vi "Set Controls.vi"(1 "Disabled Controls":refnum<vi>[](array[refnum]), 2 "Enabled Controls":refnum<vi>[](array[refnum])) -> ()   [LabVIEW 2017]
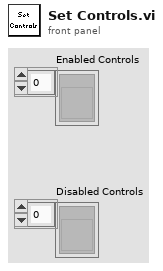
[diagram p1: front panel]
types:
  T1 = enum8{"Enabled", "Disabled", "Disabled and Grayed Out"}
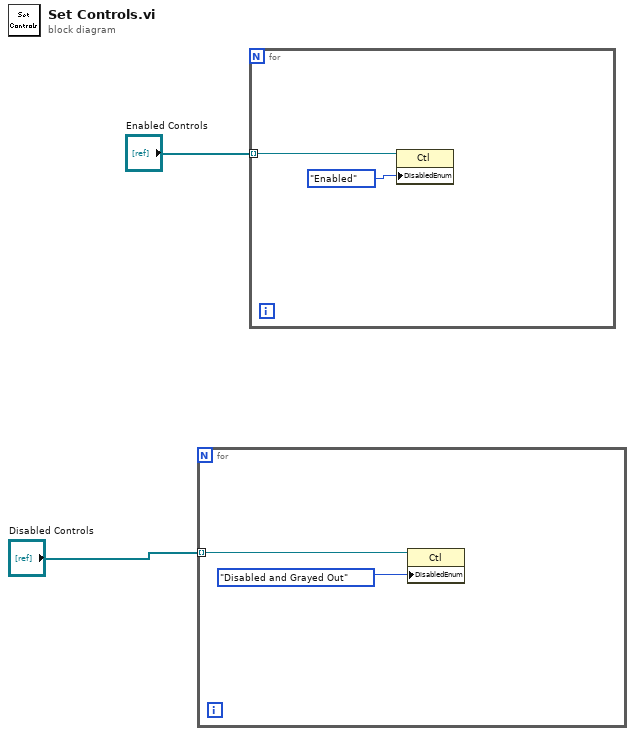
[diagram p0: block diagram]
diagram:
  n1 = for {
    tunnel: "Disabled Controls" -> [w4] mode=indexing
    n2 = property class="Ctl"(reference=w4, "DisabledEnum"=T1."Disabled and Grayed Out" ("Disabled")) -> ()  [unwired: 1 in, 2 out]
  }
  n3 = for {
    tunnel: "Enabled Controls" -> [w6] mode=indexing
    n4 = property class="Ctl"(reference=w6, "DisabledEnum"=T1."Enabled" ("Disabled")) -> ()  [unwired: 1 in, 2 out]
  }
